vi "toBoolean.vi"(8 "error in (no error)":errorcluster, 11 "Variant":variant) -> (0 "error out":errorcluster, 3 "Boolean":bool)   [LabVIEW 2018, in "Account History.lvclass"]
uses:
  Account History.lvclass
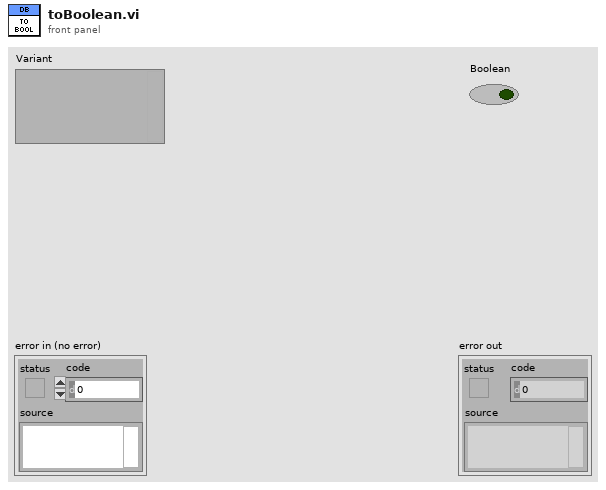
[diagram p1: front panel]
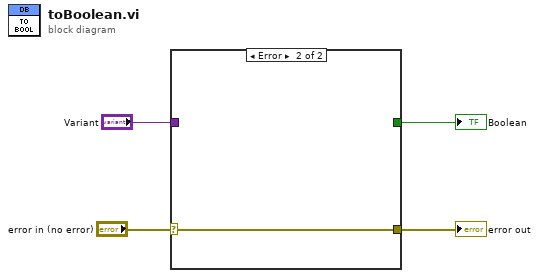
[diagram p0: block diagram]
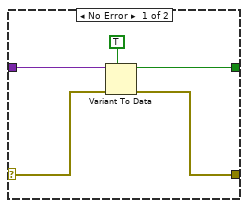
[diagram p2: hidden frame]
diagram:
  n1 = case shown="Error" "error in (no error)" {
    selector: "error in (no error)" -> [w6 w10]
    tunnel: [w5 w10] -> w3
    tunnel: "Variant" -> [w9 _]
    tunnel: [w7 _] -> w1
    frame No Error {
      n2 = Variant To Data(error in=w6, type=TRUE, Variant=w9) -> (data=w7:bool, error out=w5:errorcluster)
    }
    frame Error {
    }
  }
  "error out" <- w3
  "Boolean" <- w1
